vi "BBoxLite28A.vi"() -> ()   [LabVIEW 2017]
uses:
  C:/Users/Ivy Siao/OneDrive/NB_BackUp/Project/BBOX/BBoxLite28A_LabView_2017/BBoxAPI.dll
  BBoxAPI.dll
panel:
  out "switchChannelPower":string
  in  "Power":i32
  out "selectAAKit":i32(ring) items=["OK"=0, "WARNING"=1, "ERROR"=2, "NO_RESPONSE"=3, "ERROR_GET_SN"=10, "ERROR_DEV_TYPE"=11, "ERROR_INIT_OBJECT"=12, "ERROR_DEV_NOT_INIT"=13, "ERROR_METHOD_NOT_FOUND"=14, "ERROR_REFLECTION"=15, "ERROR_POWER"=16, "ERROR_NETWORK_NOT_INIT"=20, "ERROR_NETWORK_INIT"=21, "ERROR_NETWORK_CONNECT_TIMEOUT"=22, "ERROR_DISCONNECT"=23, "ERROR_SOCKET"=24, "ERROR_SEND_CMD"=25, "ERROR_RESP_CMD"=26, "ERROR_DEV_COUNT_ZERO"=30, "ERROR_CMD"=40, "ERROR_CMD_INIT"=41, "ERROR_BF_AAKIT"=100, "ERROR_BF_NO_AAKIT"=101, "ERROR_BF_CALI_PATH"=102, "ERROR_BF_BEAMXY"=103, "ERROR_BF_GEN"=104, "ERROR_BF_TRMODE"=105, "STATUS_BF_LOAD_CALI_INCOMPLTE"=106, "ERROR_BF_LOAD_CALI_PARSE_FAILED"=107, "ERROR_FREQ_EQUATION"=250, "ERROR_PLO_CRC"=251, "WARNING_HARMONIC"=252, "ERROR_HARMONIC_BLOCK"=253]
  out "readBeamPhaseValues":i32[][](array[numeric])
  out "readBeamGainValues":dbl[][](array[numeric])
  out "setBeamXY":i32(ring) items=["OK"=0, "WARNING"=1, "ERROR"=2, "NO_RESPONSE"=3, "ERROR_GET_SN"=10, "ERROR_DEV_TYPE"=11, "ERROR_INIT_OBJECT"=12, "ERROR_DEV_NOT_INIT"=13, "ERROR_METHOD_NOT_FOUND"=14, "ERROR_REFLECTION"=15, "ERROR_POWER"=16, "ERROR_NETWORK_NOT_INIT"=20, "ERROR_NETWORK_INIT"=21, "ERROR_NETWORK_CONNECT_TIMEOUT"=22, "ERROR_DISCONNECT"=23, "ERROR_SOCKET"=24, "ERROR_SEND_CMD"=25, "ERROR_RESP_CMD"=26, "ERROR_DEV_COUNT_ZERO"=30, "ERROR_CMD"=40, "ERROR_CMD_INIT"=41, "ERROR_BF_AAKIT"=100, "ERROR_BF_NO_AAKIT"=101, "ERROR_BF_CALI_PATH"=102, "ERROR_BF_BEAMXY"=103, "ERROR_BF_GEN"=104, "ERROR_BF_TRMODE"=105, "STATUS_BF_LOAD_CALI_INCOMPLTE"=106, "ERROR_BF_LOAD_CALI_PARSE_FAILED"=107, "ERROR_FREQ_EQUATION"=250, "ERROR_PLO_CRC"=251, "WARNING_HARMONIC"=252, "ERROR_HARMONIC_BLOCK"=253]
  in  "Angle":i32 min=-45 max=45 step=1
  in  "Beam Gain":dbl step=0.5
  out "setChannelGainPhase":string
  in  "Phase":i32 min=0 max=355 step=5
  in  "Gain":dbl step=0.5
  in  "Channel":i32=1 min=1 max=4
  in  "TxRxMode":i32=1 min=1 max=2 step=1
  out "Maxmum Gain":dbl
  out "Minimum Gain":dbl
  out "getTxRxMode":i32
  out "SwitchTxRxMode":i32(ring) items=["OK"=0, "WARNING"=1, "ERROR"=2, "NO_RESPONSE"=3, "ERROR_GET_SN"=10, "ERROR_DEV_TYPE"=11, "ERROR_INIT_OBJECT"=12, "ERROR_DEV_NOT_INIT"=13, "ERROR_METHOD_NOT_FOUND"=14, "ERROR_REFLECTION"=15, "ERROR_POWER"=16, "ERROR_NETWORK_NOT_INIT"=20, "ERROR_NETWORK_INIT"=21, "ERROR_NETWORK_CONNECT_TIMEOUT"=22, "ERROR_DISCONNECT"=23, "ERROR_SOCKET"=24, "ERROR_SEND_CMD"=25, "ERROR_RESP_CMD"=26, "ERROR_DEV_COUNT_ZERO"=30, "ERROR_CMD"=40, "ERROR_CMD_INIT"=41, "ERROR_BF_AAKIT"=100, "ERROR_BF_NO_AAKIT"=101, "ERROR_BF_CALI_PATH"=102, "ERROR_BF_BEAMXY"=103, "ERROR_BF_GEN"=104, "ERROR_BF_TRMODE"=105, "STATUS_BF_LOAD_CALI_INCOMPLTE"=106, "ERROR_BF_LOAD_CALI_PARSE_FAILED"=107, "ERROR_FREQ_EQUATION"=250, "ERROR_PLO_CRC"=251, "WARNING_HARMONIC"=252, "ERROR_HARMONIC_BLOCK"=253]
  out "setOperatingFreq":i32(ring) items=["OK"=0, "WARNING"=1, "ERROR"=2, "NO_RESPONSE"=3, "ERROR_GET_SN"=10, "ERROR_DEV_TYPE"=11, "ERROR_INIT_OBJECT"=12, "ERROR_DEV_NOT_INIT"=13, "ERROR_METHOD_NOT_FOUND"=14, "ERROR_REFLECTION"=15, "ERROR_POWER"=16, "ERROR_NETWORK_NOT_INIT"=20, "ERROR_NETWORK_INIT"=21, "ERROR_NETWORK_CONNECT_TIMEOUT"=22, "ERROR_DISCONNECT"=23, "ERROR_SOCKET"=24, "ERROR_SEND_CMD"=25, "ERROR_RESP_CMD"=26, "ERROR_DEV_COUNT_ZERO"=30, "ERROR_CMD"=40, "ERROR_CMD_INIT"=41, "ERROR_BF_AAKIT"=100, "ERROR_BF_NO_AAKIT"=101, "ERROR_BF_CALI_PATH"=102, "ERROR_BF_BEAMXY"=103, "ERROR_BF_GEN"=104, "ERROR_BF_TRMODE"=105, "STATUS_BF_LOAD_CALI_INCOMPLTE"=106, "ERROR_BF_LOAD_CALI_PARSE_FAILED"=107, "ERROR_FREQ_EQUATION"=250, "ERROR_PLO_CRC"=251, "WARNING_HARMONIC"=252, "ERROR_HARMONIC_BLOCK"=253]
  out "getFrequencyList":string[](array[string])
  out "Init":i32(ring) items=["OK"=0, "WARNING"=1, "ERROR"=2, "NO_RESPONSE"=3, "ERROR_GET_SN"=10, "ERROR_DEV_TYPE"=11, "ERROR_INIT_OBJECT"=12, "ERROR_DEV_NOT_INIT"=13, "ERROR_METHOD_NOT_FOUND"=14, "ERROR_REFLECTION"=15, "ERROR_POWER"=16, "ERROR_NETWORK_NOT_INIT"=20, "ERROR_NETWORK_INIT"=21, "ERROR_NETWORK_CONNECT_TIMEOUT"=22, "ERROR_DISCONNECT"=23, "ERROR_SOCKET"=24, "ERROR_SEND_CMD"=25, "ERROR_RESP_CMD"=26, "ERROR_DEV_COUNT_ZERO"=30, "ERROR_CMD"=40, "ERROR_CMD_INIT"=41, "ERROR_BF_AAKIT"=100, "ERROR_BF_NO_AAKIT"=101, "ERROR_BF_CALI_PATH"=102, "ERROR_BF_BEAMXY"=103, "ERROR_BF_GEN"=104, "ERROR_BF_TRMODE"=105, "STATUS_BF_LOAD_CALI_INCOMPLTE"=106, "ERROR_BF_LOAD_CALI_PARSE_FAILED"=107, "ERROR_FREQ_EQUATION"=250, "ERROR_PLO_CRC"=251, "WARNING_HARMONIC"=252, "ERROR_HARMONIC_BLOCK"=253]
  out "SN":string
  out "ScanningDevice":string[](array[string])
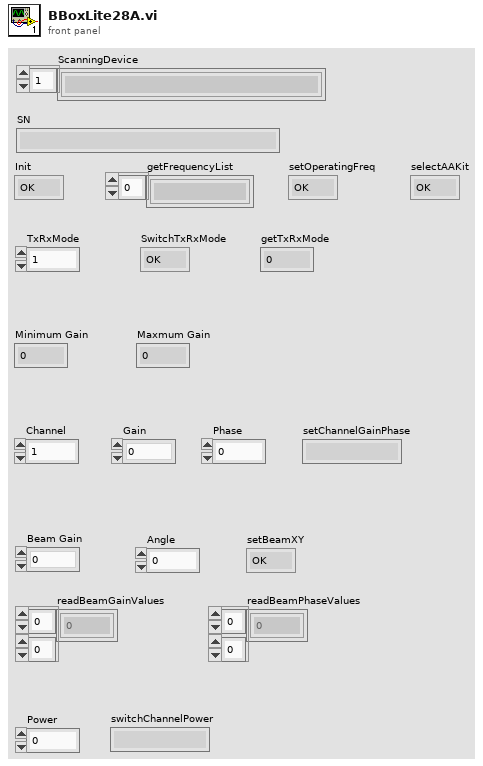
[diagram p1: front panel]
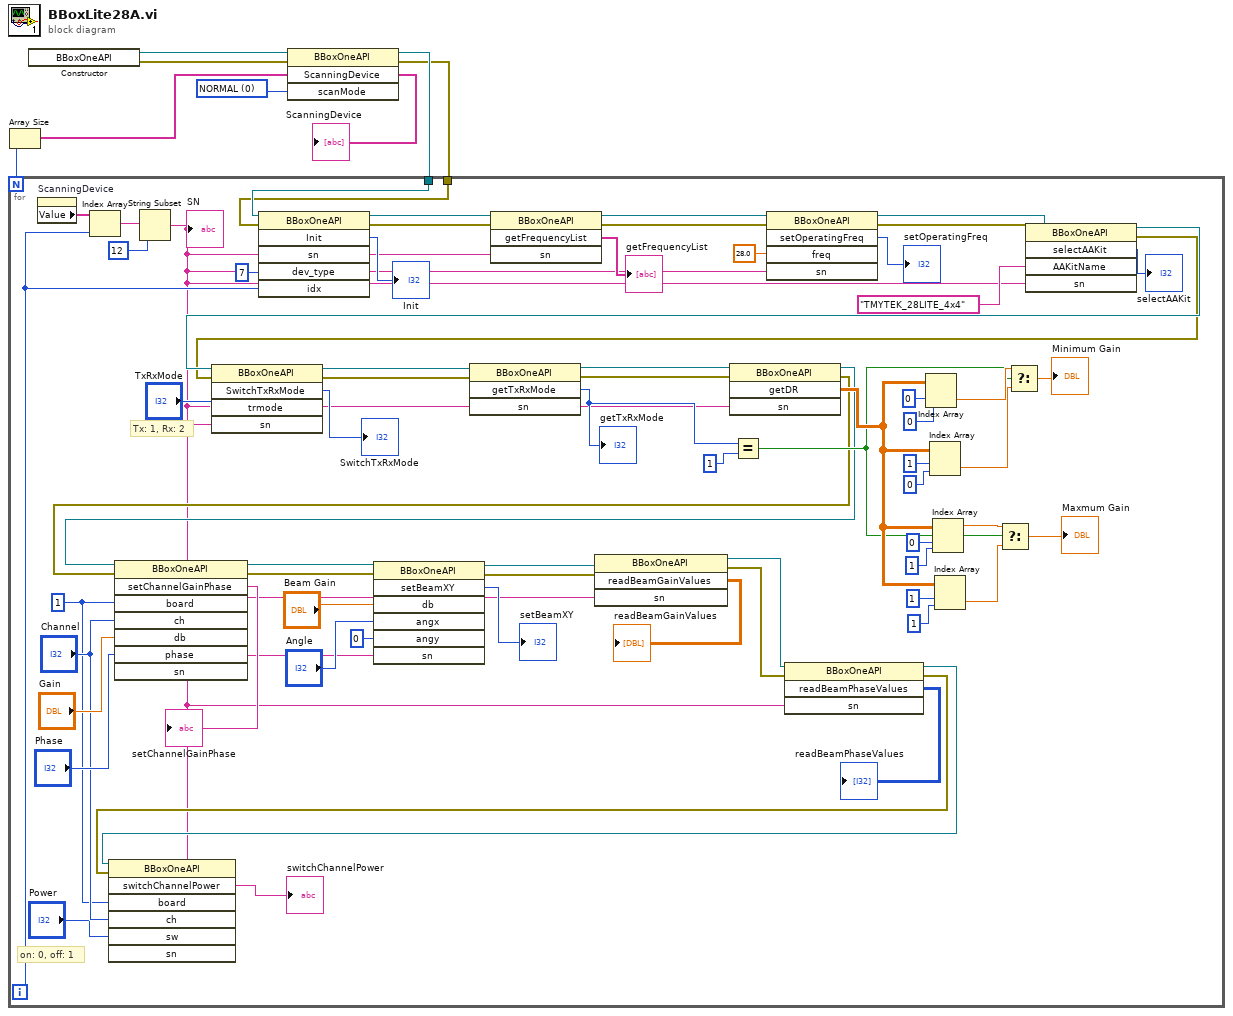
[diagram p0: block diagram]
diagram:
  w7 = 0 items=["NORMAL", "FAST"] ("scanMode")
  n1 = constructor class="BBoxOneAPI"() -> (reference out=w6:refnum<k24>, error out=w5:errorcluster)  [unwired: 3 in, 1 out]
  n2 = invoke class="BBoxOneAPI" method="ScanningDevice"(reference=w6, error in=w5, "scanMode"=w7) -> (reference out=w2:refnum<k24>, error out=w1:errorcluster, "ScanningDevice"=w3:string[])  [unwired: 1 in, 1 out]
  "ScanningDevice" <- w3
  n3 = Array Size(array=w3) -> (size(s)=w4:i32)
  n4 = for {
    N: w4 -> [_]
    tunnel: w2 -> [w73]
    tunnel: w1 -> [w72]
    i -> [w70]
    w11 = 1
    # "on: 0, off: 1"
    # "Tx: 1, Rx: 2"
    n5 = property on="ScanningDevice" class="Arr (strict)"() -> ("Value"=w76:string[])  [unwired: 2 in, 2 out]
    n6 = Index Array(array=w76, index=w70) -> (element=w75:string)
    n7 = String Subset(string=w75, length (rest)=12) -> (substring=w9:string)  [unwired: 1 in]
    "SN" <- w9
    n8 = invoke class="BBoxOneAPI" method="Init"(reference=w73, error in=w72, "sn"=w9, "dev_type"=7, "idx"=w70) -> (reference out=w68:refnum<k24>, error out=w67:errorcluster, "Init"=→"Init":i32)  [unwired: 1 in, 3 out]
    n9 = invoke class="BBoxOneAPI" method="getFrequencyList"(reference=w68, error in=w67, "sn"=w9) -> (reference out=w65:refnum<k24>, error out=w64:errorcluster, "getFrequencyList"=→"getFrequencyList":string[])  [unwired: 1 in, 1 out]
    n10 = invoke class="BBoxOneAPI" method="setOperatingFreq"(reference=w65, error in=w64, "freq"=28.0, "sn"=w9) -> (reference out=w19:refnum<k24>, error out=w20:errorcluster, "setOperatingFreq"=→"setOperatingFreq":i32)  [unwired: 1 in, 2 out]
    n11 = invoke class="BBoxOneAPI" method="selectAAKit"(reference=w19, error in=w20, "AAKitName"="TMYTEK_28LITE_4x4", "sn"=w9) -> (reference out=w18:refnum<k24>, error out=w17:errorcluster, "selectAAKit"=→"selectAAKit":i32)  [unwired: 1 in, 2 out]
    n12 = invoke class="BBoxOneAPI" method="SwitchTxRxMode"(reference=w18, error in=w17, "trmode"="TxRxMode", "sn"=w9) -> (reference out=w60:refnum<k24>, error out=w59:errorcluster, "SwitchTxRxMode"=→"SwitchTxRxMode":i32)  [unwired: 1 in, 2 out]
    n13 = invoke class="BBoxOneAPI" method="getTxRxMode"(reference=w60, error in=w59, "sn"=w9) -> (reference out=w58:refnum<k24>, error out=w57:errorcluster, "getTxRxMode"=w56:i32)  [unwired: 1 in, 1 out]
    "getTxRxMode" <- w56
    n14 = invoke class="BBoxOneAPI" method="getDR"(reference=w58, error in=w57, "sn"=w9) -> (reference out=w37:refnum<k24>, error out=w36:errorcluster, "getDR"=w45:dbl[][])  [unwired: 1 in, 1 out]
    n15 = invoke class="BBoxOneAPI" method="setChannelGainPhase"(reference=w37, error in=w36, "board"=w11, "ch"="Channel", "db"="Gain", "phase"="Phase", "sn"=w9) -> (reference out=w32:refnum<k24>, error out=w31:errorcluster, "setChannelGainPhase"=→"setChannelGainPhase":string)  [unwired: 1 in, 5 out]
    n16 = invoke class="BBoxOneAPI" method="setBeamXY"(reference=w32, error in=w31, "db"="Beam Gain", "angx"="Angle", "angy"=0, "sn"=w9) -> (reference out=w26:refnum<k24>, error out=w25:errorcluster, "setBeamXY"=→"setBeamXY":i32)  [unwired: 1 in, 4 out]
    n17 = invoke class="BBoxOneAPI" method="readBeamGainValues"(reference=w26, error in=w25, "sn"=w9) -> (reference out=w23:refnum<k24>, error out=w22:errorcluster, "readBeamGainValues"=→"readBeamGainValues":dbl[][])  [unwired: 1 in, 1 out]
    n18 = Equal?(x=w56, y=1) -> (x = y?=w42:bool)
    n19 = invoke class="BBoxOneAPI" method="readBeamPhaseValues"(reference=w23, error in=w22, "sn"=w9) -> (reference out=w14:refnum<k24>, error out=w13:errorcluster, "readBeamPhaseValues"=→"readBeamPhaseValues":i32[][])  [unwired: 1 in, 1 out]
    n20 = invoke class="BBoxOneAPI" method="switchChannelPower"(reference=w14, error in=w13, "board"=w11, "ch"="Channel", "sw"="Power", "sn"=w9) -> ("switchChannelPower"=→"switchChannelPower":string)  [unwired: 1 in, 6 out]
    n21 = Index Array(array=w45, index (row)=0, index (col)=0) -> (element=w52:dbl)
    n22 = Index Array(array=w45, index (row)=1, index (col)=0) -> (element=w49:dbl)
    n23 = Index Array(array=w45, index (row)=0, index (col)=1) -> (element=w41:dbl)
    n24 = Index Array(array=w45, index (row)=1, index (col)=1) -> (element=w40:dbl)
    n25 = Select(t=w41, s=w42, f=w40) -> (s? t:f=→"Maxmum Gain":dbl)
    n26 = Select(t=w52, s=w42, f=w49) -> (s? t:f=→"Minimum Gain":dbl)
  }
